vi "Bind To Type.vi"(8 "error in (no error)":errorcluster, 10 "Type Name":string, 11 "Known Types Binder in":refnum<class "Known Types Binder.lvclass">) -> (0 "error out":errorcluster, 2 "Type":refnum<class>, 3 "Known Types Binder out":refnum<class "Known Types Binder.lvclass">)   [LabVIEW 2017, in "Known Types Binder.lvclass"]
doc: "Controls the binding of a serialized object to a type."
uses:
  Known Types Binder.lvclass
  Known Types Binder.lvclass/Known Types Binder.ctl
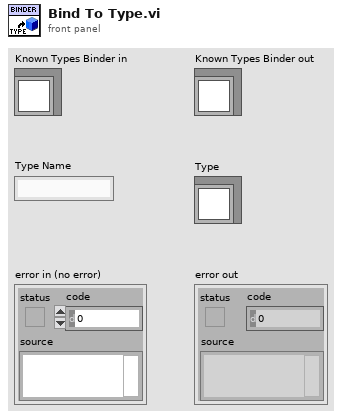
[diagram p1: front panel]
types:
  T1 = typedef "Known Types Binder.lvclass/Known Type.ctl" = cluster{"Name":string, "Type":refnum<class>}
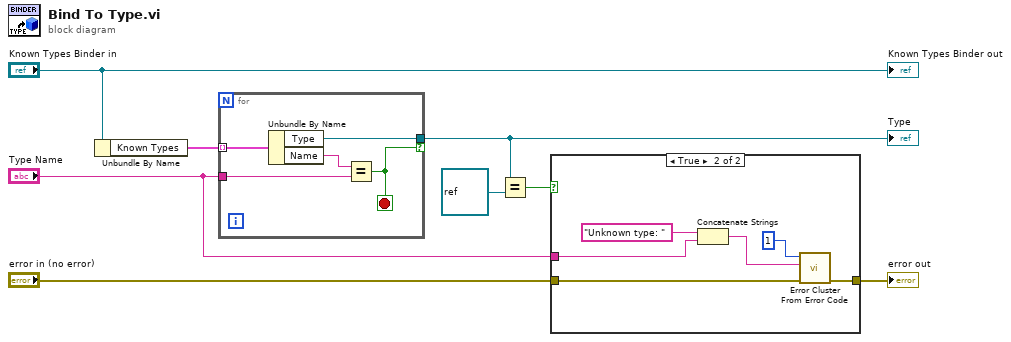
[diagram p0: block diagram]
diagram:
  n1 = Unbundle By Name("Known Types Binder in") -> ("Known Types"=w8:T1[])
  n2 = for {
    tunnel: w8 -> [w13] mode=indexing
    tunnel: "Type Name" -> [w11]
    tunnel: [w10] -> w2 if=w9
    stop <- w9 stop-if-true
    n3 = Unbundle By Name(w13) -> ("Type"=w10:refnum<class>, "Name"=w12:string)
    n4 = Equal?(x=w12, y=w11) -> (x = y?=w9:bool)
  }
  "Type" <- w2
  n5 = Equal?(x=w2, y=refnum<class> refnum) -> (x = y?=w3:bool)
  n6 = case shown="True" w3 {
    tunnel: "error in (no error)" -> [w14 w18]
    tunnel: [w14 w20] -> w1
    tunnel: "Type Name" -> [_ w16]
    frame False {
    }
    frame True {
      n7 = Concatenate Strings("Unknown type: " ("string"), w16) -> (w15:string)
      n8 = call <vilib>:"Error Cluster From Error Code.vi"("error in (no error)"=w18, "error message (\"\")"=w15, "error code (0)"=1) -> ("error out"=w20:errorcluster)  [unwired: 6 in]
    }
  }
  "error out" <- w1
  "Known Types Binder out" <- "Known Types Binder in"
